vi "Python@Script__Parameter.vi"(1 "ParamterIn":string) -> (0 "ParamterOut":string)   [LabVIEW 2019]
panel:
  in  "PythonCode":string
  in  "Confirm":bool
  # "Python@Script $PythonCode"
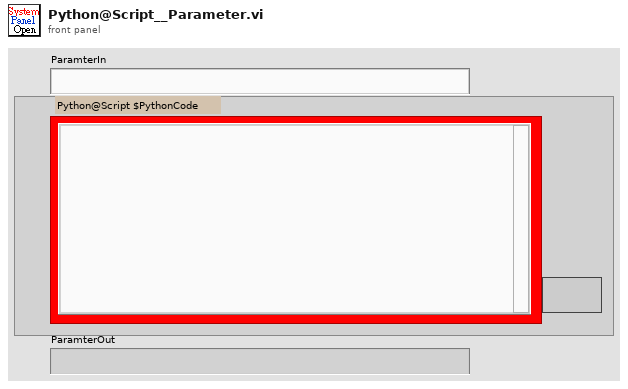
[diagram p1: front panel]
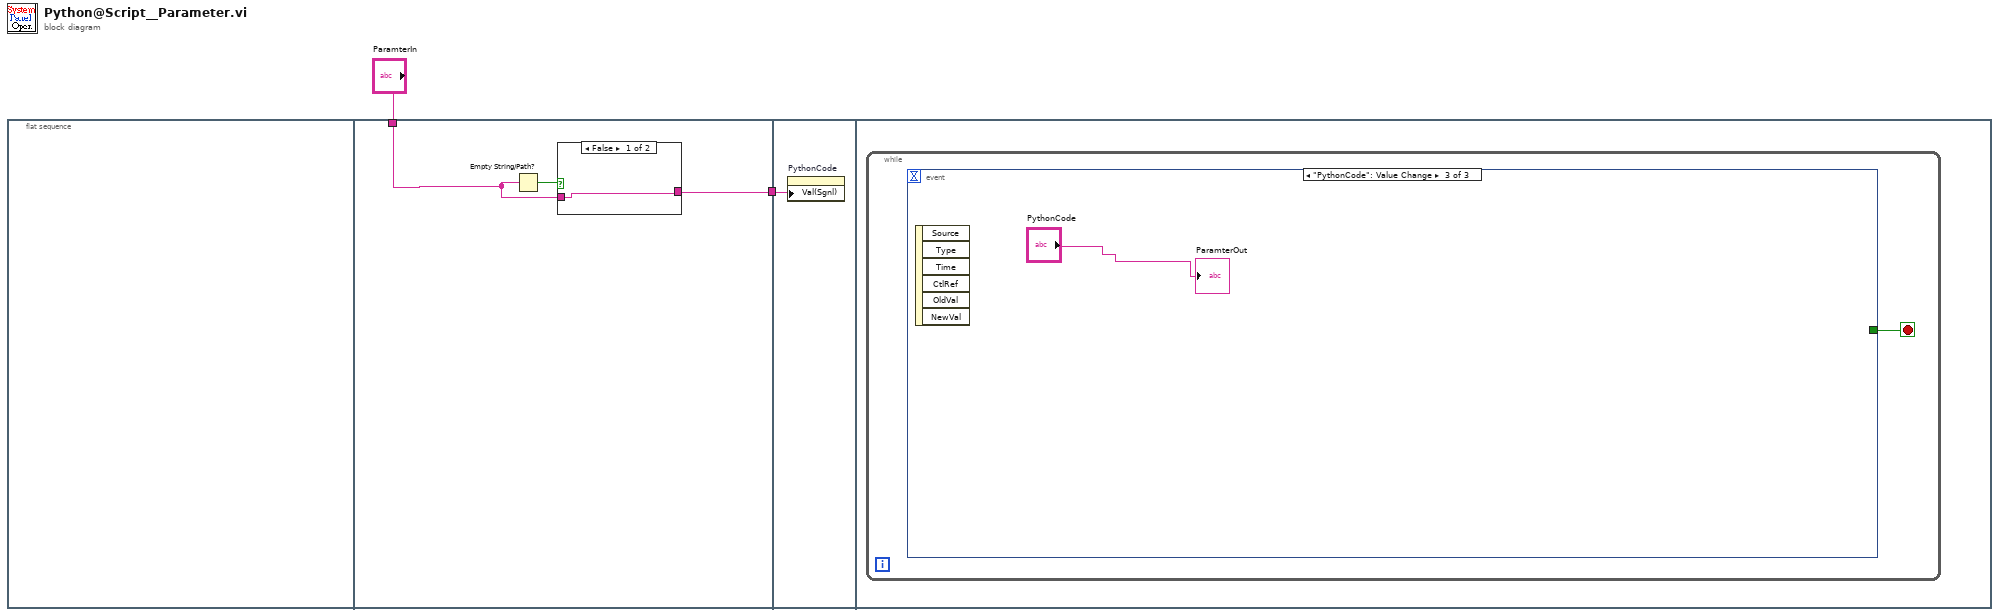
[diagram p0: block diagram]
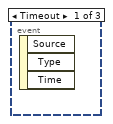
[diagram p3: hidden frame]
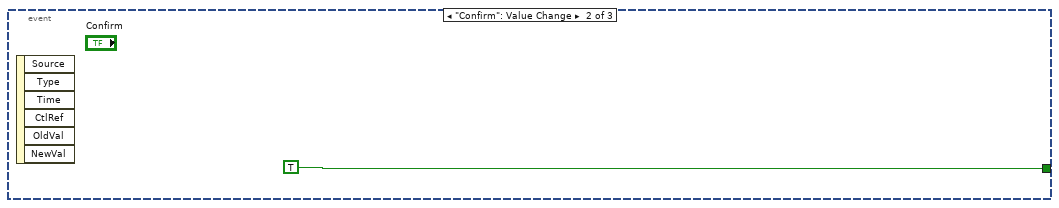
[diagram p4: hidden frame]
diagram:
  n1 = flat-sequence {
    tunnel: "ParamterIn" -> [w3]
    tunnel: [w4] -> w1
    tunnel: w1 -> [w8]
    frame #0 {
    }
    frame #1 {
      n2 = Empty String/Path?(string/path=w3) -> (empty?=w5:bool)
      n3 = case shown="False" w5 {
        tunnel: w3 -> [w6 w7]
        tunnel: [w6 w7] -> w4
        frame False {
        }
        frame True {
        }
      }
    }
    frame #2 {
      n4 = property on="PythonCode" class="Str"("Val(Sgnl)"=w8) -> ()  [unwired: 2 in, 2 out]
    }
    frame #3 {
      n5 = while {
        stop <- w9 stop-if-true
        n6 = event shown="[2] \"PythonCode\": Value Change" {
          selector: _ -> [_ _ _]
          dyn-events: _ -> [_ _ _]
          timeout: _ -> [_ _ _]
          tunnel: [_ TRUE _] -> w9
          event Timeout {
            n7 = event-data() -> ()  [unwired: 1 in, 3 out]
          }
          event "Confirm": Value Change {
            n8 = event-data() -> ()  [unwired: 1 in, 6 out]
          }
          event "PythonCode": Value Change {
            n9 = event-data() -> ()  [unwired: 1 in, 6 out]
            "ParamterOut" <- "PythonCode"
          }
        }
      }
    }
  }
